vi "util_find_owners.vi"(8 "error in (no error)":errorcluster, 11 "owner":refnum<vi>) -> (0 "error out":errorcluster, 3 "owner_name []":string[](array[string]))   [LabVIEW 2015, in "lv-build.lvlib"]
uses:
  lv-build.lvlib
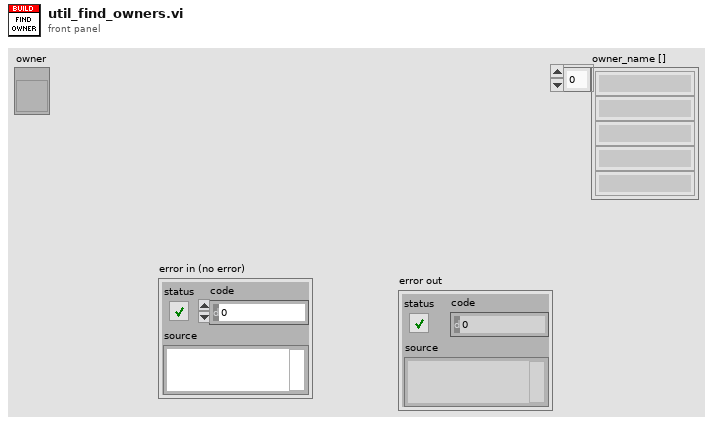
[diagram p1: front panel]
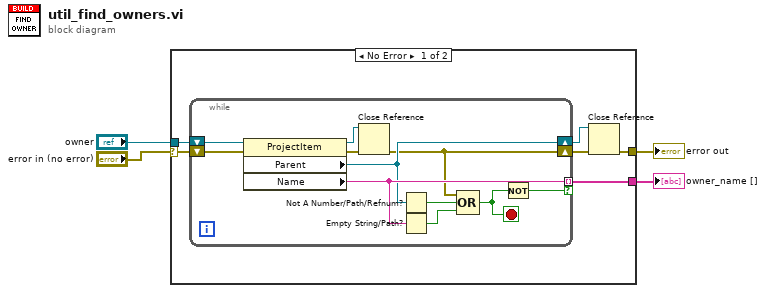
[diagram p0: block diagram]
diagram:
  n1 = case shown="No Error" "error in (no error)" {
    selector: "error in (no error)" -> [w9 w22]
    tunnel: "owner" -> [w10 _]
    tunnel: [w6 w22] -> w2
    tunnel: [w5 _] -> w1
    frame No Error {
      n2 = while {
        shift-right: [w16] -> w8
        shift-left: w10 -> [w21]
        tunnel: [w18] -> w5 mode=indexing if=w11
        shift-right: [w13] -> w7
        shift-left: w9 -> [w14]
        stop <- w12 stop-if-true
        n3 = property class="ProjectItem"(reference=w21, error in=w14) -> (reference out=w20:refnum<vi>, error out=w19:errorcluster, "Parent"=w16:refnum<vi>, "Name"=w18:string)
        n4 = Close Reference(reference=w20, error in (no error)=w19) -> (error out=w13:errorcluster)
        n5 = Not A Number/Path/Refnum?(number/path/refnum=w16) -> (NaN/Path/Refnum?=w17:bool)
        n6 = Empty String/Path?(string/path=w18) -> (empty?=w15:bool)
        n7 = Compound Arithmetic op=OR(w13, w17, w15) -> (w12:bool)
        n8 = Not(x=w12) -> (.not. x?=w11:bool)
      }
      n9 = Close Reference(reference=w8, error in (no error)=w7) -> (error out=w6:errorcluster)
    }
    frame Error {
    }
  }
  "error out" <- w2
  "owner_name []" <- w1
